vi "Example Build Array 1.vi"(8 "Error In":errorcluster) -> (0 "Error Out":errorcluster)   [LabVIEW 2018]
panel:
  out "appended array":dbl[][](array[numeric])
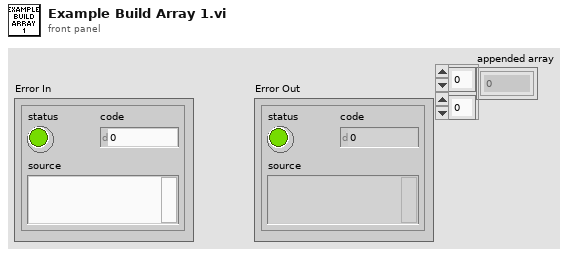
[diagram p1: front panel]
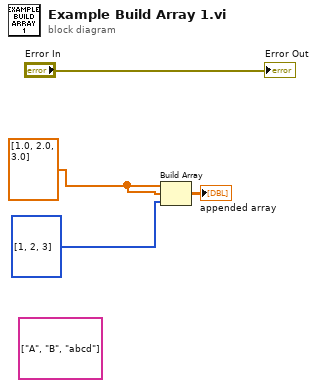
[diagram p0: block diagram]
diagram:
  (unwired) string[] ["A", "B", "abcd"]
  w2 = dbl[] [1.0, 2.0, 3.0]
  n1 = Build Array(w2, w2, i32[] [1, 2, 3]) -> (→"appended array":dbl[][])
  "Error Out" <- "Error In"
